vi "ACDC_Config_9229.vi"(8 "error in (no error)":errorcluster, 10 "Data Rate [S/s]":u32, 11 "Input Config Array":T1[](array[typedef])=[0, 0, 0, 0, 0, 0, 0, 0, 0, 0, 0, 0, 0, 0, 0, 0, 0, 0, 0, 0, 0, 0, 0, 0, 0, 0, 0, 0, 0, 0, 0, 0] items=["AC Coupled", "DC Coupled", "IEPE AC Coupled"]) -> (0 "error out":errorcluster)   [LabVIEW 2017, in "VDMS_VibAPI_8.lvlib"]
uses:
  <vilib>/addons/InsightCM/Devices/Shared/Cms/Fpga/AcquisitionFpgaTach/source/subVIs/VibAPI_8/VDMS_VibAPI_8.lvlib
  <vilib>/LabVIEW Targets/FPGA/cRIO/shared/nicrio_ModuleControls/nicrio_cRIO-9232_ConfigModeRing.ctl
  <vilib>/LabVIEW Targets/FPGA/cRIO/shared/nicrio_ModuleControls/nicrio_cRIO-9232_DataRatesRing2.ctl
  <vilib>/rvi/eio/common/nirviEmuTemplatePropertySet_errors.vi
  <vilib>/eio/EIOPropertyNode/EIOPropertyNode.xnode
  <vilib>/LabVIEW Targets/FPGA/cRIO/shared/nicrio_ModuleControls/nicrio_cRIO-9229_DataRatesRing2.ctl
  <vilib>/rvi/eio/common/nirviEmuTemplatePropertyGet_errors.vi
  <vilib>/rvi/eio/common/nirviEmuTemplatePropertyGet_noerrors.vi
  <vilib>/rvi/eio/common/nirviEmuTemplatePropertySet_noerrors.vi
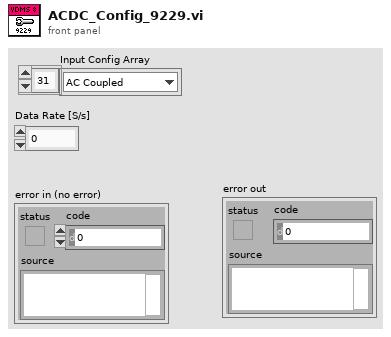
[diagram p1: front panel]
types:
  T1 = typedef "nicrio_cRIO-9232_ConfigModeRing.ctl" = u8
  T2 = typedef "nicrio_cRIO-9232_DataRatesRing2.ctl" = u8
  T3 = typedef "nicrio_cRIO-9229_DataRatesRing2.ctl" = u8
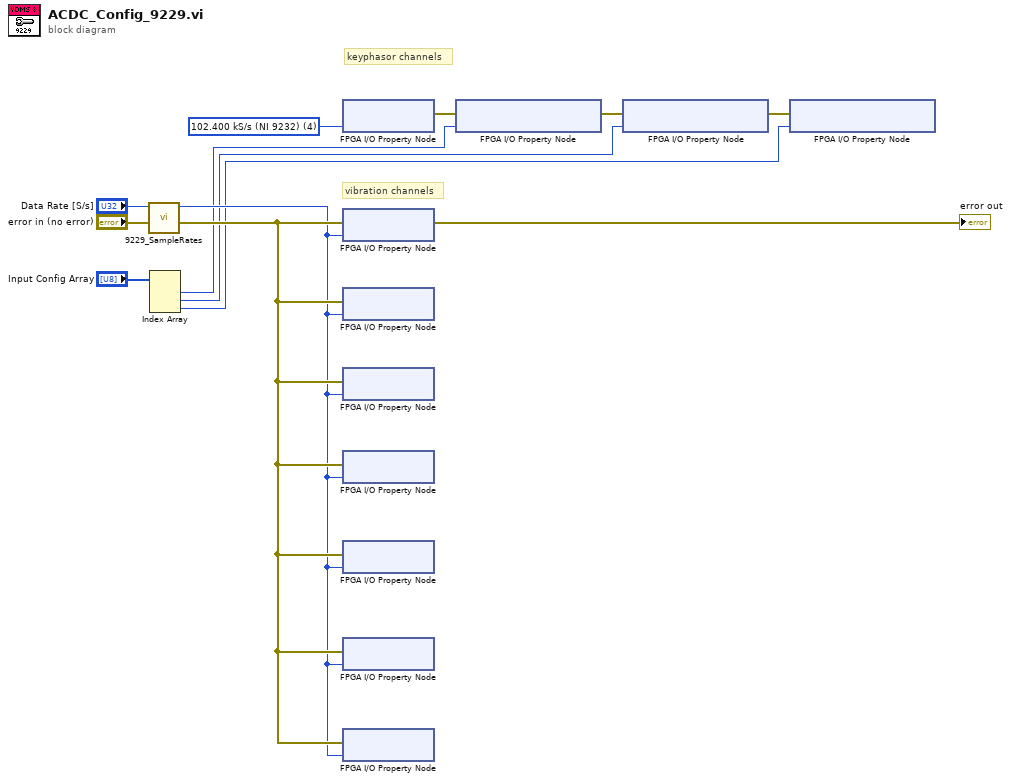
[diagram p0: block diagram]
diagram:
  w7 = T2 4 items=["102.400 kS/s (NI 9232)"=4, "51.200 kS/s (NI 9232)"=5, "34.133 kS/s (NI 9232)"=12, "25.600 kS/s (NI 9232)"=6, "20.480 kS/s (NI 9232)"=20, "17.067 kS/s (NI 9232)"=13, "14.629 kS/s (NI 9232)"=28, "12.800 kS/s (NI 9232)"=10, "11.378 kS/s (NI 9232)"=36, "10.240 kS/s (NI 9232)"=21, "9.309 kS/s (NI 9232)"=44, "8.533 kS/s (NI 9232)"=14, "7.877 kS/s (NI 9232)"=52, "7.314 kS/s (NI 9232)"=29, "6.827 kS/s (NI 9232)"=60, "6.400 kS/s (NI 9232)"=18, "6.024 kS/s (NI 9232)"=68, "5.689 kS/s (NI 9232)"=37, "5.389 kS/s (NI 9232)"=76, "5.120 kS/s (NI 9232)"=22, "4.876 kS/s (NI 9232)"=84, "4.655 kS/s (NI 9232)"=45, "4.452 kS/s (NI 9232)"=92, "4.267 kS/s (NI 9232)"=26, "4.096 kS/s (NI 9232)"=100, "3.938 kS/s (NI 9232)"=53, "3.657 kS/s (NI 9232)"=30, "3.413 kS/s (NI 9232)"=61, "3.200 kS/s (NI 9232)"=34, "3.012 kS/s (NI 9232)"=69, "2.844 kS/s (NI 9232)"=38, "2.695 kS/s (NI 9232)"=77, "2.560 kS/s (NI 9232)"=42, "2.438 kS/s (NI 9232)"=85, "2.327 kS/s (NI 9232)"=46, "2.226 kS/s (NI 9232)"=93, "2.133 kS/s (NI 9232)"=50, "2.048 kS/s (NI 9232)"=101, "1.969 kS/s (NI 9232)"=54, "1.829 kS/s (NI 9232)"=58, "1.707 kS/s (NI 9232)"=62, "1.600 kS/s (NI 9232)"=66, "1.506 kS/s (NI 9232)"=70, "1.422 kS/s (NI 9232)"=74, "1.347 kS/s (NI 9232)"=78, "1.280 kS/s (NI 9232)"=82, "1.219 kS/s (NI 9232)"=86, "1.164 kS/s (NI 9232)"=90, "1.113 kS/s (NI 9232)"=94, "1.067 kS/s (NI 9232)"=98, "1.024 kS/s (NI 9232)"=102, "0.985 kS/s (NI 9232)"=106] ("Data Rate")
  # "vibration channels"
  # "keyphasor channels"
  n1 = call <vilib>:"9229_SampleRates.vi"("error in (no error)"="error in (no error)", "Data Rate [S/s]"="Data Rate [S/s]") -> ("error out"=w11:errorcluster, "Data Rate"=w6:T3)  [unwired: 8 in]
  n2 = Index Array(array="Input Config Array") -> (element #1=w4:T1, element #2=w3:T1, element #3=w2:T1)  [unwired: 3 in]
  n3 = xnode "FPGA I/O Property Node"("Data Rate"=w7) -> ("error out"=w10:errorcluster)  [unwired: 2 in, 1 out]
  n4 = xnode "FPGA I/O Property Node"("error in"=w11, "Data Rate"=w6) -> ("error out"=→"error out":errorcluster)  [unwired: 1 in, 1 out]
  n5 = xnode "FPGA I/O Property Node"("error in"=w11, "Data Rate"=w6) -> ()  [unwired: 1 in, 2 out]
  n6 = xnode "FPGA I/O Property Node"("error in"=w11, "Data Rate"=w6) -> ()  [unwired: 1 in, 2 out]
  n7 = xnode "FPGA I/O Property Node"("error in"=w11, "Data Rate"=w6) -> ()  [unwired: 1 in, 2 out]
  n8 = xnode "FPGA I/O Property Node"("error in"=w11, "Data Rate"=w6) -> ()  [unwired: 1 in, 2 out]
  n9 = xnode "FPGA I/O Property Node"("error in"=w11, "Data Rate"=w6) -> ()  [unwired: 1 in, 2 out]
  n10 = xnode "FPGA I/O Property Node"("error in"=w11, "Data Rate"=w6) -> ()  [unwired: 1 in, 2 out]
  n11 = xnode "FPGA I/O Property Node"("error in"=w10, "Input Configuration"=w4) -> ("error out"=w9:errorcluster)  [unwired: 1 in, 1 out]
  n12 = xnode "FPGA I/O Property Node"("error in"=w9, "Input Configuration"=w3) -> ("error out"=w8:errorcluster)  [unwired: 1 in, 1 out]
  n13 = xnode "FPGA I/O Property Node"("error in"=w8, "Input Configuration"=w2) -> ()  [unwired: 1 in, 2 out]
